vi "GDSString_ParsePropertyMethod.vi"(11 "PropertyMethodContent":string) -> (2 "SetProperty":T1, 3 "GetProperty":T1)   [LabVIEW 2016]
uses:
  <resource>/Framework/Providers/Open_GDS/ClassProviders/Common/CommonVIs/CommonVIs_PropertyType.ctl
  <resource>/Framework/Providers/Open_GDS/ClassProviders/Common/String/GDSString_AccessScopeModifierType.ctl
panel:
  # "get\n\t{\n\t    // We don't allow this to be used on Friday.\n\t    if (this._day == DayOfWeek.Friday)\n\t    {\n\t\tthrow new Exception(\"Invalid access\");\n\t    }\n\t    return this._day;\n\t}\n\tset\n\t{\n\t    this._day = value;\n\t}"
  # "get\n\t{\n\t    return this._number;\n\t}\n\tset\n\t{\n\t    this._number = value;\n\t}"
  # "public int Id\n    {\n\tget;\n\tprivate set;\n    }"
  # "public double Hours\n    {\n        get { return seconds / 3600; }\n        set { seconds = value * 3600; }\n    }"
  # "{ get { ... } set { ... }"
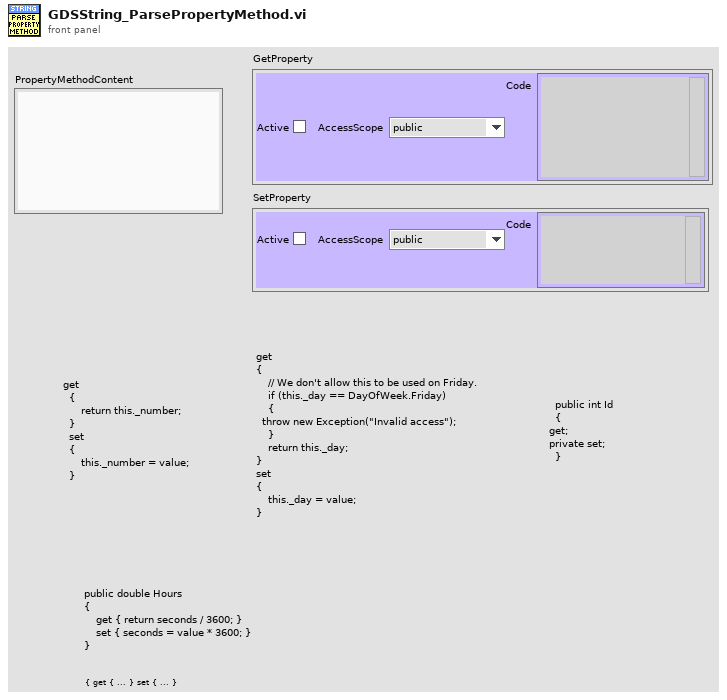
[diagram p1: front panel]
types:
  T1 = typedef "CommonVIs_PropertyType.ctl" = cluster{"Active":bool, "AccessScope":T2, "Code":string}
  T2 = typedef "GDSString_AccessScopeModifierType.ctl" = enum16{"public", "private", "protected", "internal"}
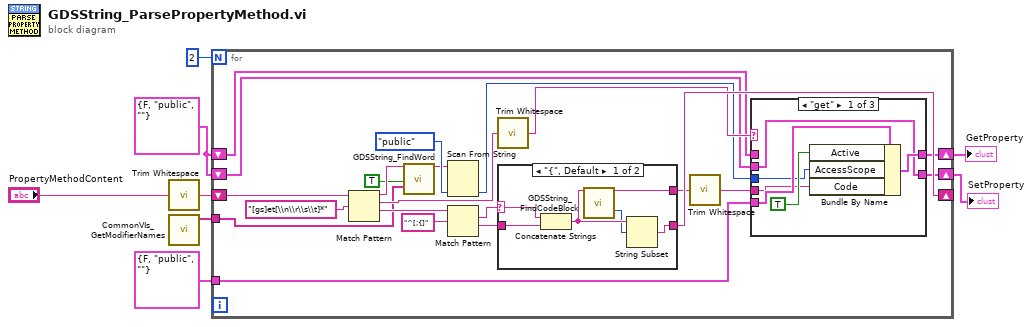
[diagram p0: block diagram]
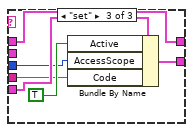
[diagram p3: hidden frame]
diagram:
  w4 = T1 {"Active"=FALSE, "AccessScope"=enum."public", "Code"=""} ("GetProperty")
  n1 = call <vilib>:"Trim Whitespace.vi"("string"="PropertyMethodContent") -> ("trimmed string"=w7:string)  [unwired: 1 in]
  n2 = call <resource>:"CommonVIs_GetModifierNames.vi"() -> ("AccessScopeModifiers"=w1:string[])  [unwired: 9 in, 2 out]
  n3 = for {
    N: 2 -> [_]
    shift-right: [w24] -> _
    shift-left: w7 -> [w27]
    tunnel: T1 {"Active"=FALSE, "AccessScope"=enum."public", "Code"=""} ("GetProperty") -> [w21]
    shift-right: [w20] -> w3
    shift-left: w4 -> [w19]
    shift-right: [w18] -> w2
    shift-left: w4 -> [w17]
    tunnel: w1 -> [w14]
    n4 = Match Pattern(string=w27, regular expression="[gs]et[\\n\\r\\s\\t]*") -> (before substring=w15:string, match substring=w23:string, after substring=w29:string)  [unwired: 1 in, 1 out]
    n5 = call <resource>:"GDSString_FindWord.vi"("Text"=w15, "Search Backwards"=TRUE, "AllowedWords(PatternMatching)"=w14) -> ("NextWord"=w11:string)  [unwired: 11 in, 5 out]
    n6 = Scan From String(input string=w11, default 1=GDSString_AccessScopeModifierType."public" ("AccessScope")) -> (output 1=w10:T2)  [unwired: 3 in, 3 out]
    n7 = Match Pattern(string=w29, regular expression="^[;{]") -> (match substring=w26:string, after substring=w25:string)  [unwired: 1 in, 2 out]
    n8 = call <vilib>:"Trim Whitespace.vi"("string"=w23) -> ("trimmed string"=w22:string)  [unwired: 1 in]
    n9 = case shown="\"{\", Default" w26 {
      selector: w26 -> [w50 _]
      tunnel: w25 -> [w49 w51]
      tunnel: [w45 w51] -> w24
      tunnel: [w48 _] -> w16
      frame "{", Default {
        n10 = Concatenate Strings(w50, w49) -> (w47:string)
        n11 = call <resource>:"GDSString_FindCodeBlock.vi"("Text"=w47) -> ("BlockText"=w48:string, "BlockEnd(Outside)"=w46:i32)  [unwired: 10 in, 7 out]
        n12 = String Subset(string=w47, offset (0)=w46) -> (substring=w45:string)  [unwired: 1 in]
      }
      frame ";" {
      }
    }
    n13 = call <vilib>:"Trim Whitespace.vi"("string"=w16) -> ("trimmed string"=w9:string)  [unwired: 1 in]
    n14 = case shown="\"get\"" w22 {
      tunnel: w21 -> [w36 _ w42]
      tunnel: [w34 w37 w44] -> w20
      tunnel: w19 -> [_ w37 w44]
      tunnel: [w33 w38 w41] -> w18
      tunnel: w17 -> [w33 w38 _]
      tunnel: w9 -> [w32 _ w40]
      tunnel: w10 -> [w31 _ w39]
      frame "get" {
        n15 = Bundle By Name(cluster=w36, "Active"=TRUE, "AccessScope"=w31, "Code"=w32) -> (w34:T1)
      }
      frame Default {
      }
      frame "set" {
        n16 = Bundle By Name(cluster=w42, "Active"=TRUE, "AccessScope"=w39, "Code"=w40) -> (w41:T1)
      }
    }
  }
  "SetProperty" <- w2
  "GetProperty" <- w3
